vi "colores_letras.vi"(8 "error in (no error)":errorcluster, 11 "Image 2":T1(plugin-control)) -> (0 "error out":errorcluster, 1 "String (OCR/OCV 1)":string, 2 "Classes (Color Classification 1)":string[](array[string]))   [LabVIEW 2020, in "Analisis.lvlib"]
uses:
  Analisis.lvlib
  <vilib>/vision/Classification.llb/IMAQ Classifier Read Options.ctl
  <vilib>/vision/NI_Vision_Development_Module.lvlib
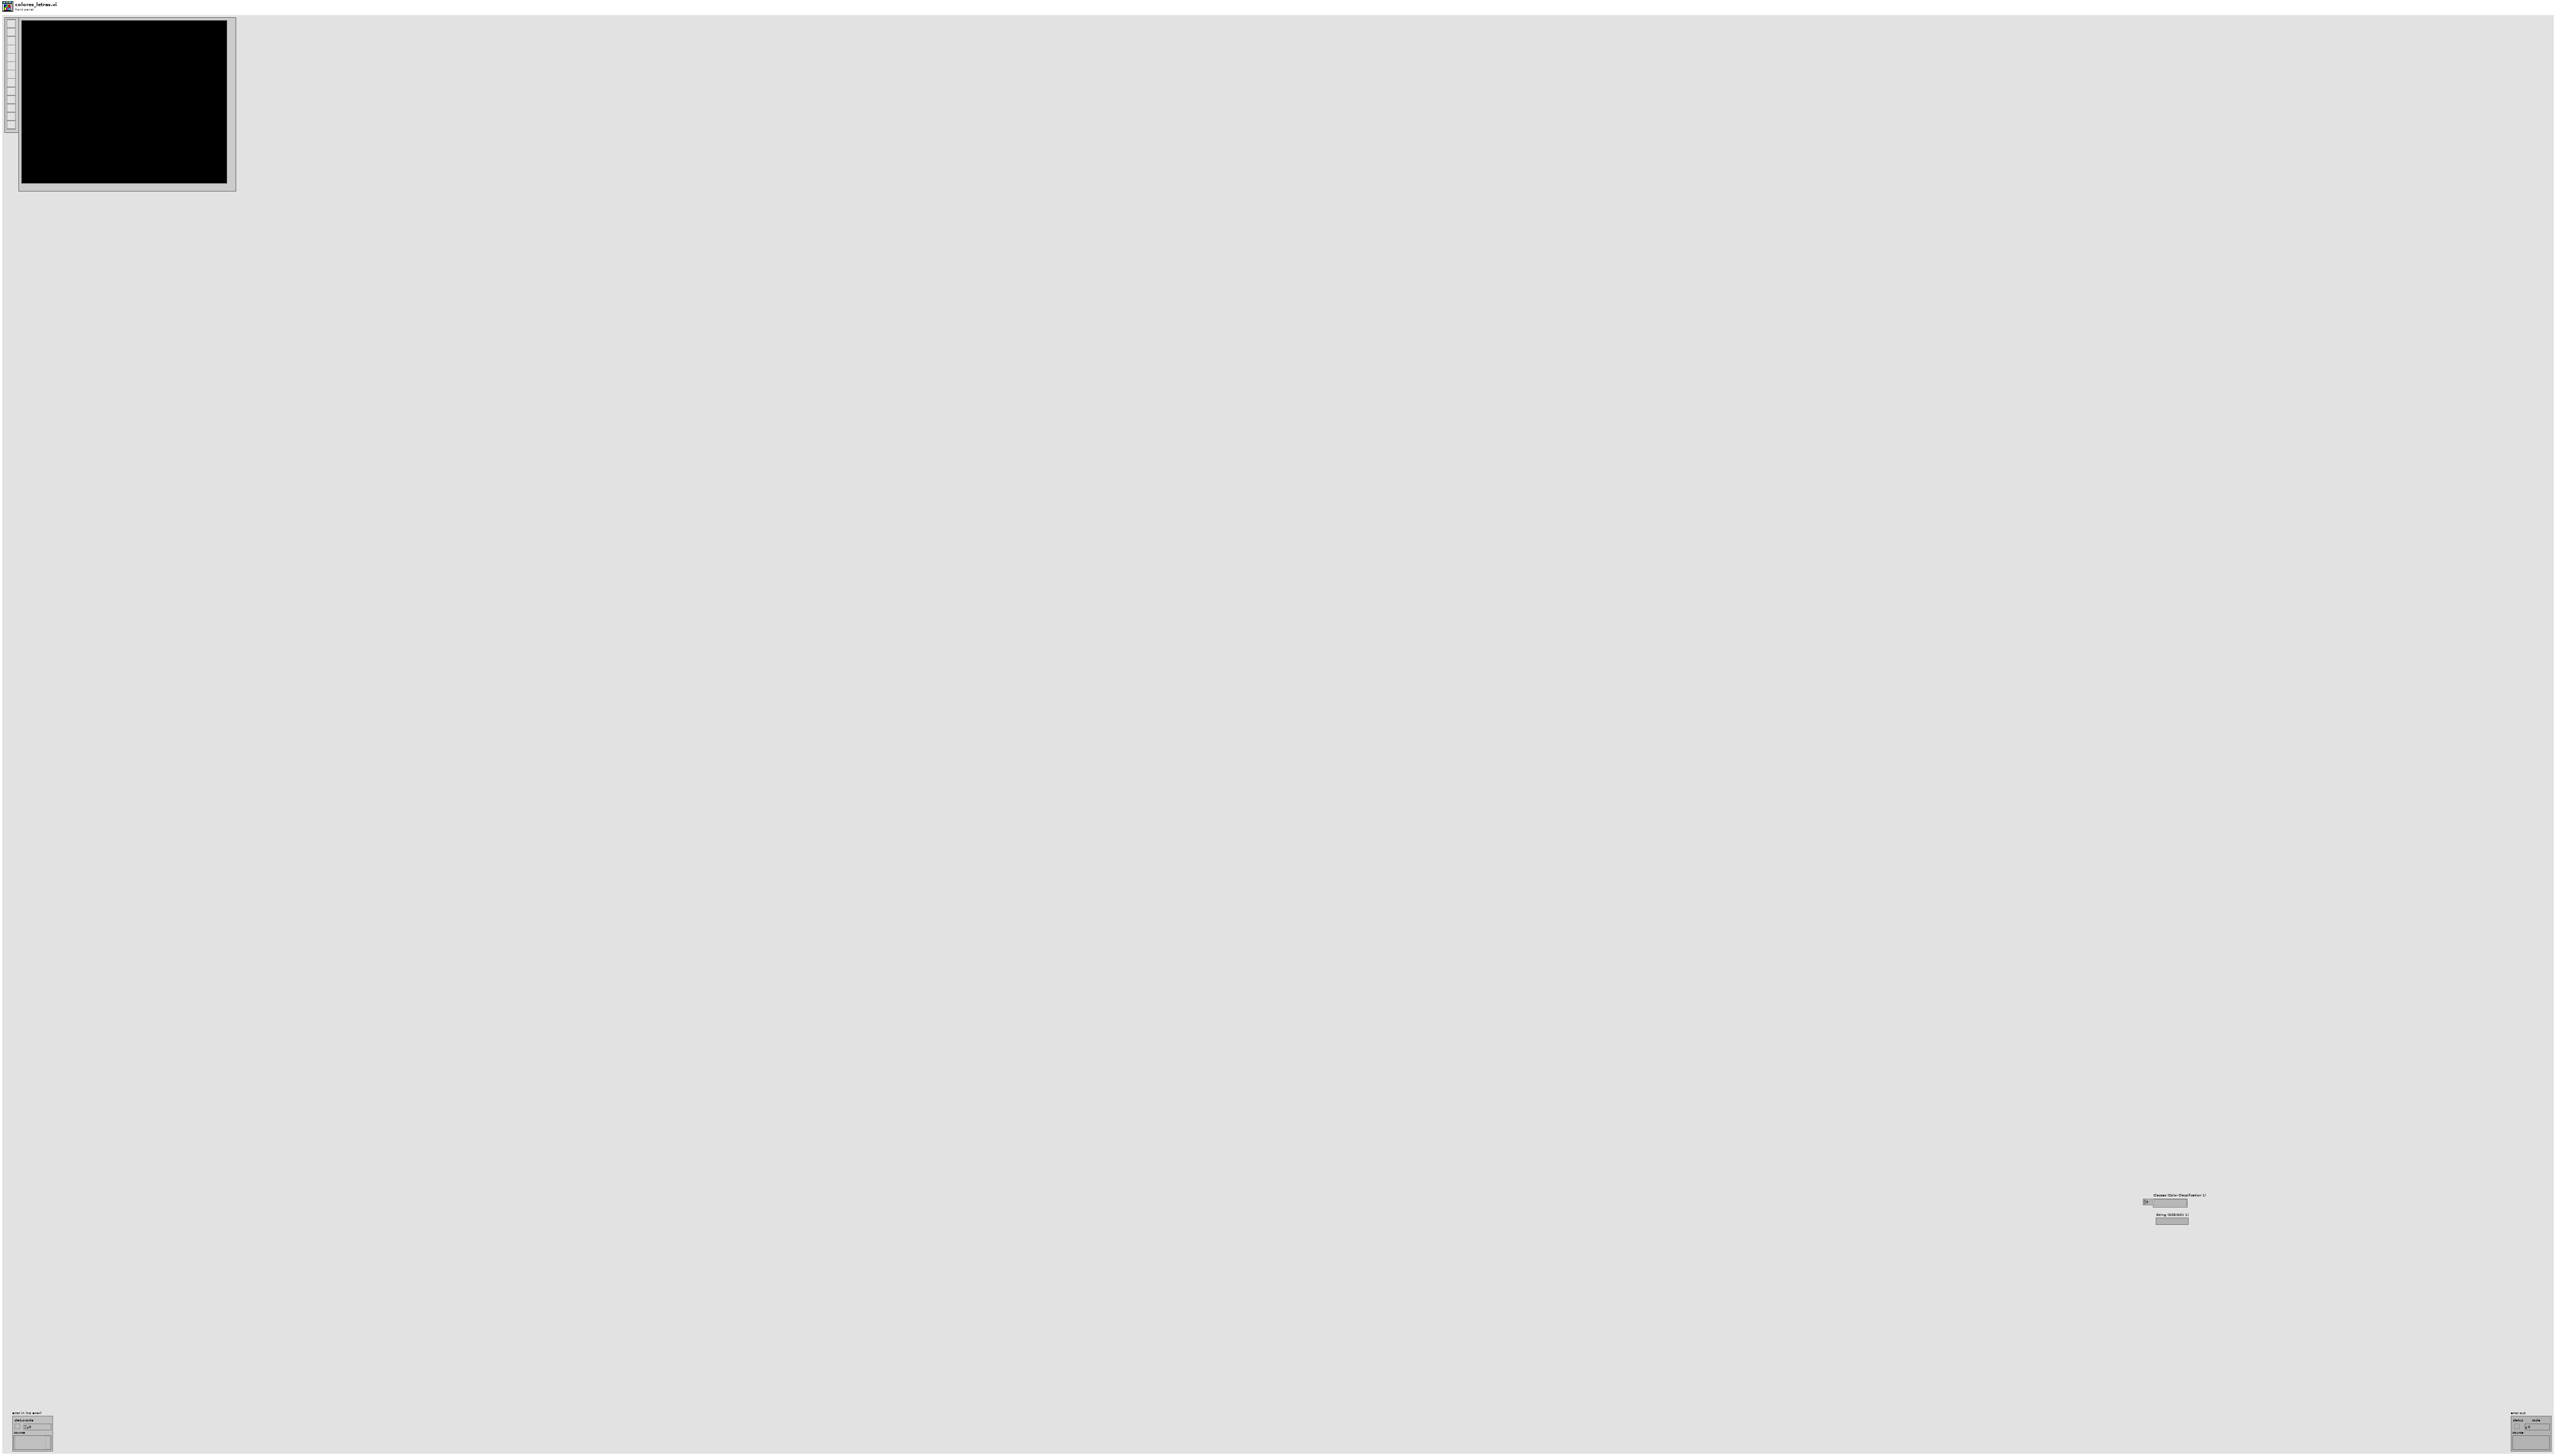
[diagram p1: front panel]
types:
  T1 = typedef "IMAQ Image.ctl" = refnum<image>
  T2 = cluster{"Threshold Data":cluster{"Method":enum16{"Fixed Range", "Uniform", "Linear", "Non Linear", "Local", "Color"}, "Looking for":u32, "Color Mode":u32, "Kernel Size":cluster{"Width":i32, "Height":i32}, "Ranges":cluster{"Min":i32, "Max":i32}[]}, "Reject Border":bool, "Number Of Erosions":i32, "Size & Spacing":cluster{"Segment Algorithm":u16, "Min Bounding Rect Width":i32, "Max Bounding Rect Width":i32, "Min Bounding Rect Height":i32, "Max Bounding Rect Height":i32, "Min Character Size":i32, "Max Character Size":i32, "Min Char Spacing":i32, "Max Horiz Element Spacing":i32, "Max Vert Element Spacing":i32, "Max Space Distance":i32}, "Read Options":cluster{"Read Strategy":i32, "Read Resolution":i32, "Scale Dependant":bool, "Aspect Ratio":i32, "Acceptance Level":i32, "Substitution Character":string, "MultiLine":bool}, "Valid Characters":cluster{"Pre-defined characters":i32, "User-defined characters":string}[], "Use Text Pattern":bool, "Orientation":u32, "# Lines Expected":u32, "Number of Blocks":i32}
  T3 = cluster{"Global Rectangle":i32[], "Contours":cluster{"ID":enum32{"External", "Internal"}, "Type":u32, "Coordinates":i32[]}[]}
  T4 = typedef "IMAQ Classifier Read Options.ctl" = i32
  T5 = typedef "IMAQ Classifier Session.ctl" = refnum<k1>
  T6 = typedef "ROI Descriptor" = cluster{"Global Rectangle":i32[], "Contours":cluster{"ID":enum32{"External", "Internal"}, "Type":u32, "Coordinates":i32[]}[]}
  T7 = typedef "IMAQ OCR Session.ctl" = refnum<k1>
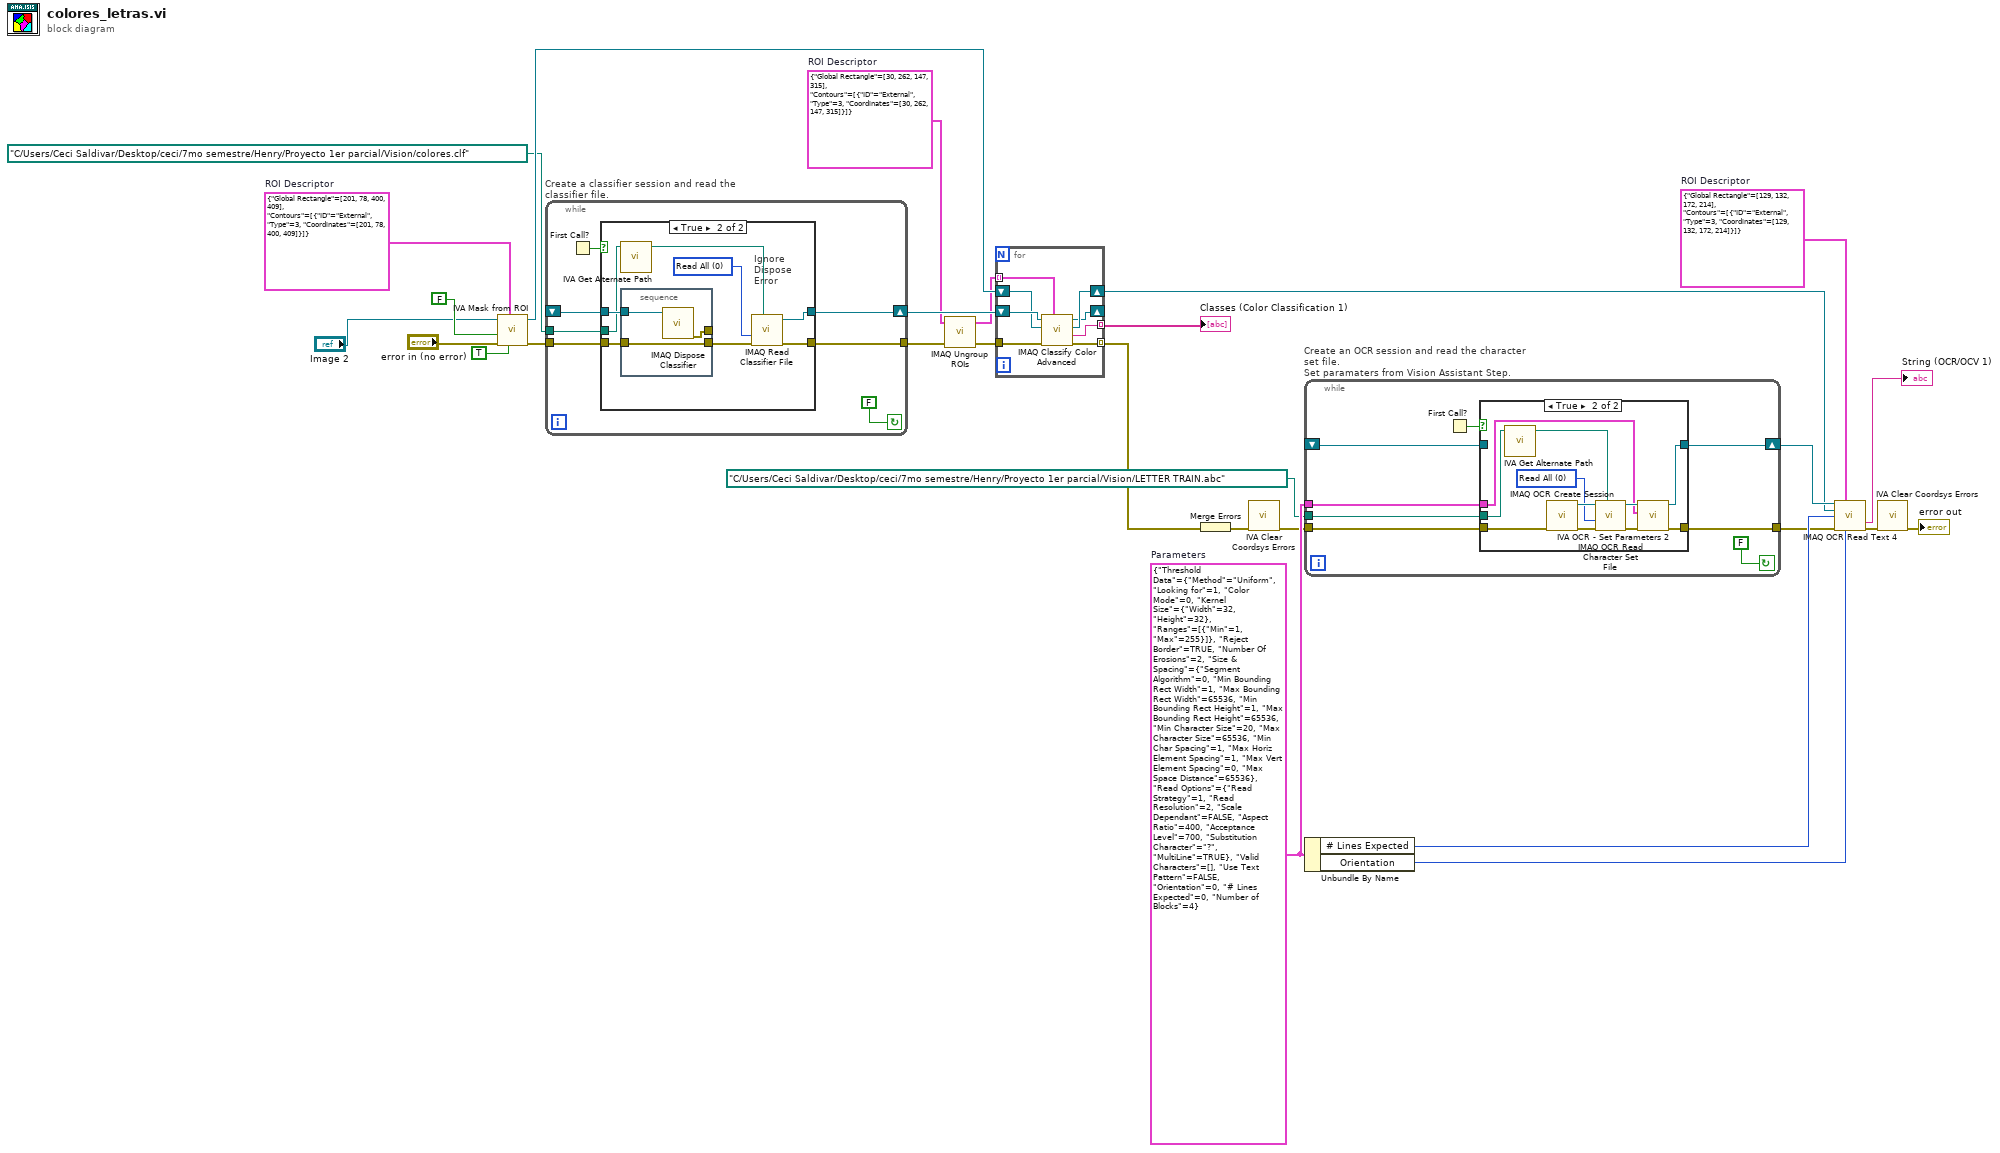
[diagram p0: block diagram]
diagram:
  w22 = T2 {"Threshold Data"={"Method"=enum."Uniform", "Looking for"=1, "Color Mode"=0, "Kernel Size"={"Width"=32, "Height"=32}, "Ranges"=[{"Min"=1, "Max"=255}]}, "Reject Border"=TRUE, "Number Of Erosions"=2, "Size & Spacing"={"Segment Algorithm"=0, "Min Bounding Rect Width"=1, "Max Bounding Rect Width"=65536, "Min Bounding Rect Height"=1, "Max Bounding Rect Height"=65536, "Min Character Size"=20, "Max Character Size"=65536, "Min Char Spacing"=1, "Max Horiz Element Spacing"=1, "Max Vert Element Spacing"=0, "Max Space Distance"=65536}, "Read Options"={"Read Strategy"=1, "Read Resolution"=2, "Scale Dependant"=FALSE, "Aspect Ratio"=400, "Acceptance Level"=700, "Substitution Character"="?", "MultiLine"=TRUE}, "Valid Characters"=[], "Use Text Pattern"=FALSE, "Orientation"=0, "# Lines Expected"=0, "Number of Blocks"=4}  # Parameters
  w20 = T3 {"Global Rectangle"=[129, 132, 172, 214], "Contours"=[{"ID"=enum."External", "Type"=3, "Coordinates"=[129, 132, 172, 214]}]}  # ROI Descriptor
  w9 = T3 {"Global Rectangle"=[30, 262, 147, 315], "Contours"=[{"ID"=enum."External", "Type"=3, "Coordinates"=[30, 262, 147, 315]}]}  # ROI Descriptor
  w3 = T3 {"Global Rectangle"=[201, 78, 400, 409], "Contours"=[{"ID"=enum."External", "Type"=3, "Coordinates"=[201, 78, 400, 409]}]}  # ROI Descriptor
  n1 = call <vilib>:"IVA Mask from ROI.vi"("Shrink"=TRUE, "ROI Descriptor"=w3, "error in (no error)"="error in (no error)", "Out / In"=FALSE, "Image Src"="Image 2") -> ("error out"=w6:errorcluster, "Image Out"=w16:T1)  [unwired: 5 out]
  n2 = while "Create a classifier session and read the classifier file." {
    shift-right: [w35] -> w17
    shift-left: _ -> [w34]
    tunnel: w6 -> [w32]
    tunnel: [w31] -> w10
    tunnel: path "C:/Users/Ceci Saldivar/Desktop/ceci/7mo semestre/Henry/Proyecto 1er parcial/Vision/colores.clf" ("File Path") -> [w30]
    stop <- FALSE continue-if-true
    n3 = First Call?() -> (First Call?: T/F=w29:bool)
    n4 = case shown="True" w29 {
      tunnel: [w37 w44] -> w35
      tunnel: w34 -> [w37 w42]
      tunnel: w32 -> [w36 w41]
      tunnel: [w36 w43] -> w31
      tunnel: w30 -> [_ w39]
      frame False {
      }
      frame True {
        w45 = T4 0 items=["Read All", "Add Samples, Do Not Change Options", "Read Options, Do Not Add Samples"] ("Read Options")
        # "Ignore Dispose Error"
        n5 = call <vilib>:"IVA Get Alternate Path.vi"("Path In"=w39) -> ("Path Out"=w38:path)  [unwired: 10 out]
        n6 = stacked-sequence {
          tunnel: w42 -> [w48]
          tunnel: w41 -> [w47]
          tunnel: [w47] -> w40
          tunnel: [w46] -> _
          frame #0 {
            n7 = call "IMAQ Dispose Classifier"("Classifier Session"=w48) -> ("error out"=w46:errorcluster)  [unwired: 1 in, 9 out]
          }
        }
        n8 = call "IMAQ Read Classifier File"("File Path"=w38, "error in (no error)"=w40, "Read Options"=w45) -> ("error out"=w43:errorcluster, "Classifier Session"=w44:T5)  [unwired: 1 in, 6 out]
      }
    }
  }
  n9 = call "IMAQ Ungroup ROIs"("error in (no error)"=w10, "ROI Descriptor"=w9) -> ("error out"=w11:errorcluster, "ROI Descriptors out"=w12:T6[])  [unwired: 2 out]
  n10 = for {
    tunnel: [w56] -> w8 mode=indexing
    tunnel: [w55] -> w13 mode=indexing
    tunnel: w11 -> [w53]
    tunnel: w12 -> [w52] mode=indexing
    shift-right: [w50] -> w21
    shift-left: w16 -> [w51]
    shift-right: [w49] -> _
    shift-left: w17 -> [w54]
    n11 = call "IMAQ Classify Color Advanced"("ROI Descriptor"=w52, "error in (no error)"=w53, "Image"=w51, "Classifier Session"=w54) -> ("error out"=w55:errorcluster, "Class"=w56:string, "Image (dup)"=w50:T1, "Classifier Session (dup)"=w49:T5)  [unwired: 4 out]
  }
  "Classes (Color Classification 1)" <- w8
  n12 = Merge Errors(w13) -> (w14:errorcluster)
  n13 = call <vilib>:"IVA Clear Coordsys Errors.vi"("error in (no error)"=w14) -> ("error out"=w15:errorcluster)  [unwired: 10 in]
  n14 = while "Create an OCR session and read the character set file.\nSet paramaters from Vision Assistant Step." {
    shift-right: [w61] -> w24
    shift-left: _ -> [w60]
    tunnel: w15 -> [w63]
    tunnel: w22 -> [w59]
    tunnel: path "C:/Users/Ceci Saldivar/Desktop/ceci/7mo semestre/Henry/Proyecto 1er parcial/Vision/LETTER TRAIN.abc" ("File Path") -> [w58]
    tunnel: [w57] -> w23
    stop <- FALSE continue-if-true
    n15 = First Call?() -> (First Call?: T/F=w62:bool)
    n16 = case shown="True" w62 {
      tunnel: w58 -> [_ w70]
      tunnel: w63 -> [w65 w74]
      tunnel: [w66 w72] -> w61
      tunnel: [w65 w71] -> w57
      tunnel: w59 -> [_ w67]
      tunnel: w60 -> [w66 _]
      frame False {
      }
      frame True {
        w75 = 0 items=["Read All", "Read Character Set Only", "Read Properties Only"] ("Read Options")
        n17 = call <vilib>:"IVA Get Alternate Path.vi"("Path In"=w70) -> ("Path Out"=w69:path)  [unwired: 10 out]
        n18 = call "IMAQ OCR Create Session"("error in (no error)"=w74) -> ("error out"=w76:errorcluster, "IMAQ OCR Session"=w77:T7)  [unwired: 9 out]
        n19 = call "IMAQ OCR Read Character Set File"("File Path"=w69, "error in (no error)"=w76, "Read Options"=w75, "IMAQ OCR Session"=w77) -> ("error out"=w73:errorcluster, "IMAQ OCR Session (dup)"=w68:T7)  [unwired: 1 in, 5 out]
        n20 = call <vilib>:"IVA OCR - Set Parameters 2.vi"("error in (no error)"=w73, "Parameters"=w67, "IMAQ OCR Session"=w68) -> ("error out"=w71:errorcluster, "IMAQ OCR Session Out"=w72:T7)  [unwired: 7 in]
      }
    }
  }
  n21 = Unbundle By Name(w22) -> ("# Lines Expected"=w26:u32, "Orientation"=w25:u32)
  n22 = call "IMAQ OCR Read Text 4"("IMAQ OCR Session"=w24, "ROI Descriptor"=w20, "Image"=w21, "Number of Lines Requested"=w26, "error in (no error)"=w23, "Orientation"=w25) -> ("Read String"=→"String (OCR/OCV 1)":string, "error out"=w27:errorcluster)  [unwired: 8 out]
  n23 = call <vilib>:"IVA Clear Coordsys Errors.vi"("error in (no error)"=w27) -> ("error out"=→"error out":errorcluster)  [unwired: 10 in]
